vi "Write Replot request.vi"(8 "error in (no error)":errorcluster, 10 "Replot request":bool, 11 "Plot in":refnum<class "Plot.lvclass">) -> (0 "error out":errorcluster, 3 "Plot out":refnum<class "Plot.lvclass">)   [LabVIEW 2018, in "Plot.lvclass"]
uses:
  Plot.lvclass
  Plot.lvclass/Plot.ctl
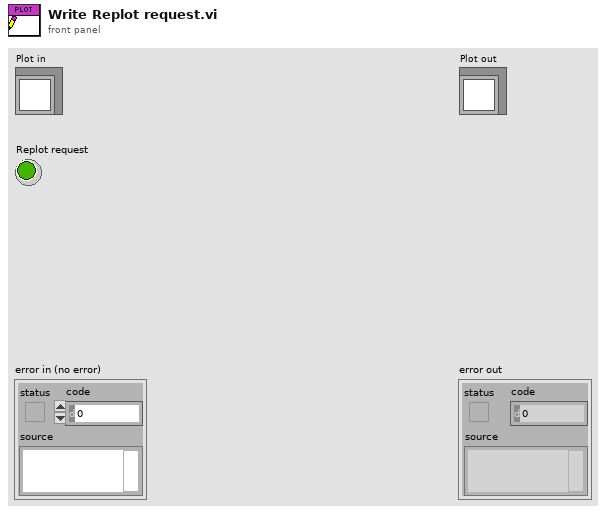
[diagram p1: front panel]
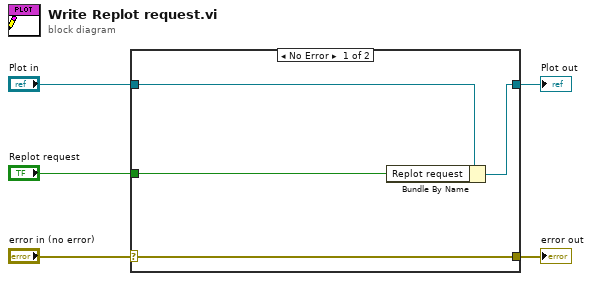
[diagram p0: block diagram]
diagram:
  n1 = case shown="No Error" "error in (no error)" {
    selector: "error in (no error)" -> [w9 w10]
    tunnel: [w9 w10] -> w4
    tunnel: [w7 w11] -> w2
    tunnel: "Plot in" -> [w8 w11]
    tunnel: "Replot request" -> [w6 _]
    frame No Error {
      n2 = Bundle By Name(cluster=w8, "Replot request"=w6) -> (w7:refnum<class "Plot.lvclass">)
    }
    frame Error {
    }
  }
  "error out" <- w4
  "Plot out" <- w2
